vi "CMD-ME record.vi"() -> ()   [LabVIEW 2020]
uses:
  <vilib>/Instr/_visa.llb/VISA Configure Serial Port (Instr).vi
panel:
  out "String":string
  in  "baud rate (38400)":u32=9600
  in  "COM Port":refnum<visa-resource-name>
  in  "Stop":bool
  in  "Start":bool
  # "Records data from CMD-ME / Geoprospectors Version"
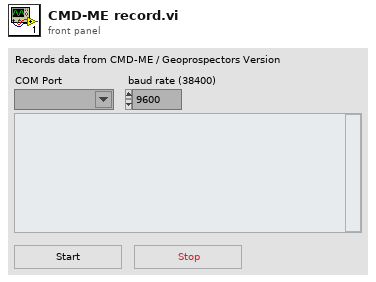
[diagram p1: front panel]
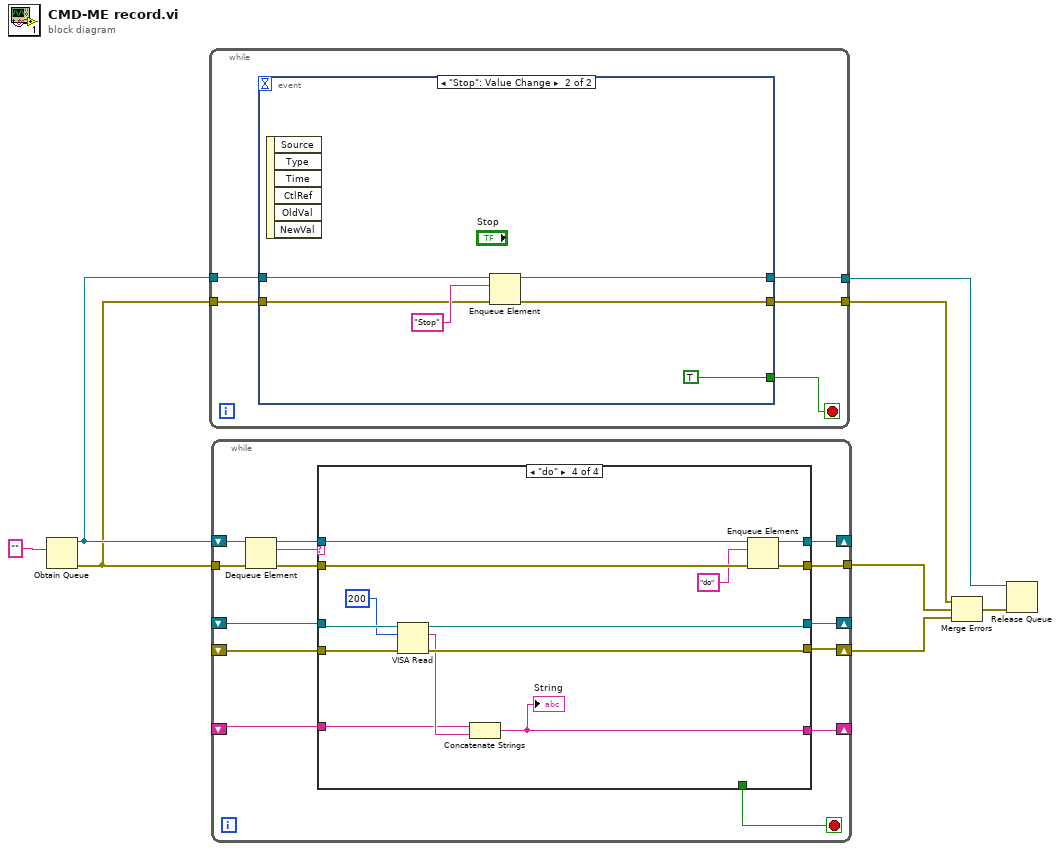
[diagram p0: block diagram]
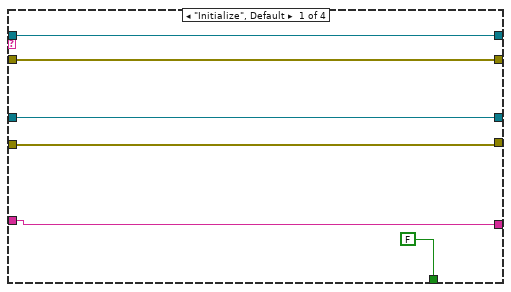
[diagram p2: hidden frame]
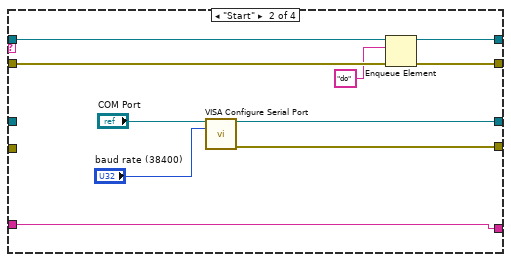
[diagram p3: hidden frame]
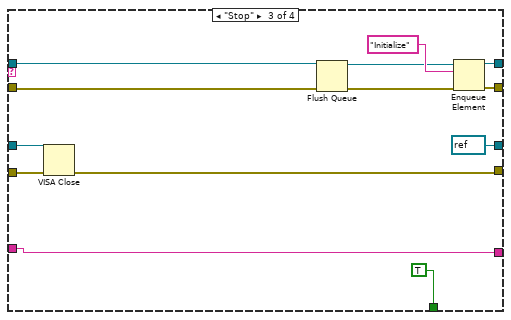
[diagram p4: hidden frame]
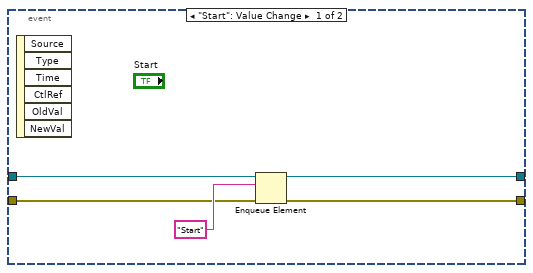
[diagram p5: hidden frame]
diagram:
  n1 = Obtain Queue(element data type="") -> (queue out=w8:refnum<queue>, error out=w6:errorcluster)  [unwired: 4 in, 1 out]
  n2 = while {
    tunnel: w8 -> [w13]
    tunnel: [w12] -> w1
    tunnel: w6 -> [w11]
    tunnel: [w10] -> w3
    stop <- w9 stop-if-true
    n3 = event shown="[1] \"Stop\": Value Change" {
      selector: _ -> [_ _]
      dyn-events: _ -> [_ _]
      timeout: _ -> [_ _]
      tunnel: w13 -> [w18 w24]
      tunnel: [w17 w22] -> w12
      tunnel: w11 -> [w15 w20]
      tunnel: [w14 w19] -> w10
      tunnel: [_ TRUE] -> w9
      event "Start": Value Change {
        n4 = event-data() -> ()  [unwired: 1 in, 6 out]
        n5 = Enqueue Element(queue=w18, element="Start", error in (no error)=w15) -> (queue out=w17:refnum<queue>, error out=w14:errorcluster)  [unwired: 1 in, 1 out]
      }
      event "Stop": Value Change {
        n6 = event-data() -> ()  [unwired: 1 in, 6 out]
        n7 = Enqueue Element(queue=w24, element="Stop", error in (no error)=w20) -> (queue out=w22:refnum<queue>, error out=w19:errorcluster)  [unwired: 1 in, 1 out]
      }
    }
  }
  n8 = while {
    shift-right: [w36] -> _
    shift-left: _ -> [w34]
    shift-right: [w35] -> w5
    shift-left: _ -> [w33]
    tunnel: [w29] -> w4
    shift-right: [w30] -> _
    shift-left: w8 -> [w38]
    tunnel: w6 -> [w28]
    shift-right: [w25] -> _
    shift-left: _ -> [w26]
    stop <- w27 stop-if-true
    n9 = Dequeue Element(queue=w38, error in (no error)=w28) -> (queue out=w32:refnum<queue>, element=w37:string, error out=w31:errorcluster)  [unwired: 1 in, 1 out]
    n10 = case shown="\"do\"" w37 {
      tunnel: [w42 w52 refnum<visa-resource-name> refnum ("VISA resource name out") w72] -> w36
      tunnel: [w41 w51 w62 w71] -> w35
      tunnel: w34 -> [w42 _ w63 w74]
      tunnel: w33 -> [w41 _ w64 w75]
      tunnel: w32 -> [w44 w49 w56 w80]
      tunnel: w31 -> [w43 w50 w57 w79]
      tunnel: [w44 w48 w67 w78] -> w30
      tunnel: [w43 w47 w66 w77] -> w29
      tunnel: [FALSE _ TRUE _] -> w27
      tunnel: w26 -> [w39 w45 w55 w69]
      tunnel: [w39 w45 w55 w68] -> w25
      frame "Initialize", Default {
      }
      frame "Start" {
        n11 = call-poly "VISA Configure Serial Port"("VISA resource name"="COM Port", "baud rate (9600)"="baud rate (38400)") -> ("VISA resource name out"=w52:refnum<visa-resource-name>, "error out"=w51:errorcluster)  [unwired: 12 in]
        n12 = Enqueue Element(queue=w49, element="do", error in (no error)=w50) -> (queue out=w48:refnum<queue>, error out=w47:errorcluster)  [unwired: 1 in, 1 out]
      }
      frame "Stop" {
        n13 = VISA Close(VISA resource name=w63, error in (no error)=w64) -> (error out=w62:errorcluster)
        n14 = Flush Queue(queue=w56, error in (no error)=w57) -> (queue out=w59:refnum<queue>, error out=w58:errorcluster)  [unwired: 1 out]
        n15 = Enqueue Element(queue=w59, element="Initialize", error in (no error)=w58) -> (queue out=w67:refnum<queue>, error out=w66:errorcluster)  [unwired: 1 in, 1 out]
      }
      frame "do" {
        n16 = VISA Read(VISA resource name=w74, byte count=200, error in (no error)=w75) -> (VISA resource name out=w72:refnum<visa-resource-name>, read buffer=w70:string, error out=w71:errorcluster)  [unwired: 1 out]
        n17 = Concatenate Strings(w69, w70) -> (w68:string)
        "String" <- w68
        n18 = Enqueue Element(queue=w80, element="do", error in (no error)=w79) -> (queue out=w78:refnum<queue>, error out=w77:errorcluster)  [unwired: 1 in, 1 out]
      }
    }
  }
  n19 = Merge Errors(w3, w4, w5) -> (w2:errorcluster)
  n20 = Release Queue(queue=w1, error in (no error)=w2) -> ()  [unwired: 1 in, 3 out]
